vi "Write pdoBufferSize.vi"(8 "error in (no error)":errorcluster, 10 "pdoBufferSize":u16=10, 11 "MotorControllerClass in":refnum<class "MotorControllerClass.lvclass">) -> (0 "error out":errorcluster, 3 "MotorControllerClass out":refnum<class "MotorControllerClass.lvclass">)   [LabVIEW 2018, in "MotorControllerClass.lvclass"]
uses:
  BMS/MotorControllerClass.lvclass
  BMS/MotorControllerClass.lvclass/MotorControllerClass.ctl
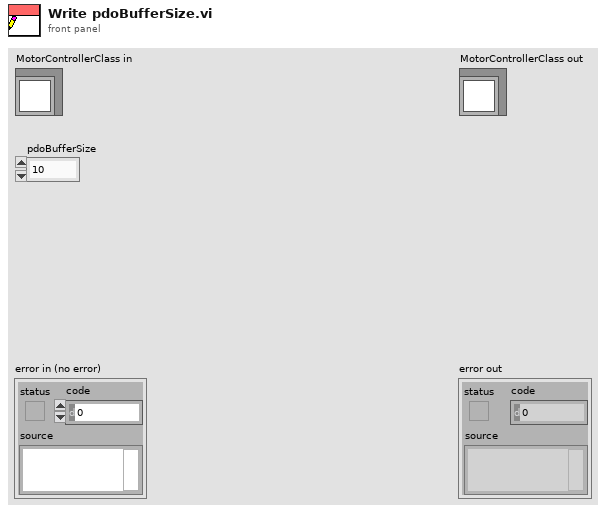
[diagram p1: front panel]
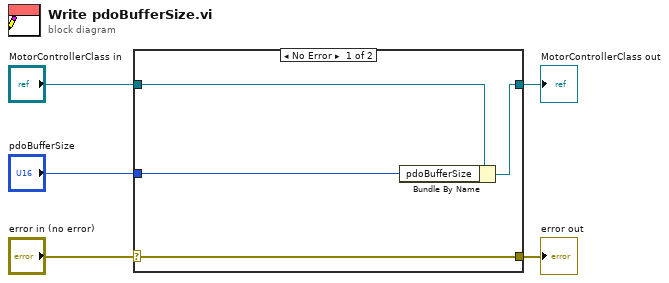
[diagram p0: block diagram]
diagram:
  n1 = case shown="No Error" "error in (no error)" {
    selector: "error in (no error)" -> [w9 w10]
    tunnel: [w9 w10] -> w4
    tunnel: [w7 w11] -> w2
    tunnel: "MotorControllerClass in" -> [w8 w11]
    tunnel: "pdoBufferSize" -> [w6 _]
    frame No Error {
      n2 = Bundle By Name(cluster=w8, "pdoBufferSize"=w6) -> (w7:refnum<class "MotorControllerClass.lvclass">)
    }
    frame Error {
    }
  }
  "error out" <- w4
  "MotorControllerClass out" <- w2
